vi "Shooting Equation.vi"(10 "Object Y":dbl, 11 "Shoot Equation Parameter Array":dbl[](array[numeric])) -> (3 "Output":dbl)   [LabVIEW 2016]
uses:
  <vilib>/Rock Robotics/Network Tables/NT Read Number.vi
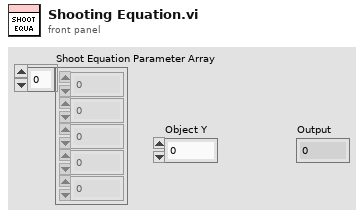
[diagram p1: front panel]
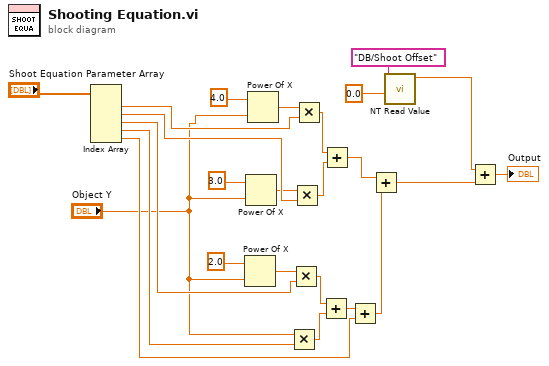
[diagram p0: block diagram]
diagram:
  n1 = Index Array(array="Shoot Equation Parameter Array") -> (element #1=w17:dbl, element #2=w18:dbl, element #3=w19:dbl, element #4=w20:dbl, element #5=w21:dbl)  [unwired: 5 in]
  n2 = Power Of X(1:"Object Y", 2:2.0 ("x")) -> (0:w7:dbl)
  n3 = Power Of X(1:"Object Y", 2:3.0 ("x")) -> (0:w5:dbl)
  n4 = Power Of X(1:"Object Y", 2:4.0 ("x")) -> (0:w3:dbl)
  n5 = Multiply(x="Object Y", y=w20) -> (x*y=w11:dbl)
  n6 = Multiply(x=w7, y=w19) -> (x*y=w10:dbl)
  n7 = Multiply(x=w5, y=w18) -> (x*y=w9:dbl)
  n8 = Multiply(x=w3, y=w17) -> (x*y=w8:dbl)
  n9 = Add(x=w10, y=w11) -> (x+y=w12:dbl)
  n10 = Add(x=w8, y=w9) -> (x+y=w14:dbl)
  n11 = Add(x=w12, y=w21) -> (x+y=w13:dbl)
  n12 = Add(x=w14, y=w13) -> (x+y=w24:dbl)
  n13 = call-poly <vilib>:"NT Read Value.vi"("Default Value"=0.0, "Name"="DB/Shoot Offset") -> ("Numeric"=w25:dbl)  [unwired: 8 in, 1 out]
  n14 = Add(x=w25, y=w24) -> (x+y=→"Output":dbl)
